vi "modbusTxLoop.vi"(11 "Modbus Port Settings":T1) -> ()   [LabVIEW 2015]
uses:
  DataTypes/ModbusPortSettings.ctl
  DataTypes/TxLoopData.ctl
  DataTypes/TxStates.ctl
  <vilib>/Platform/TimedLoop/XDataNode/timing_clust.ctl
  <vilib>/Platform/TimedLoop/XDataNode/nitl_modes.ctl
  <vilib>/Platform/TimedLoop/XDataNode/wakeup.ctl
  Telemetry/DataTypes/TelemetryUpdateMode.ctl
  <vilib>/rvi/Emulation/niFpgaSctlEmulationGetInTimedLoop.vi
  <vilib>/rvi/Emulation/niFpgaEmulationReportErrorSimple.vi
  <vilib>/rvi/Emulation/niFpgaGetClockAttributes.vi
  <vilib>/rvi/Emulation/niFpgaCriticalErrorInLSC.vi
  <vilib>/rvi/Emulation/niFpgaEmulationIsFPGAContextNoSignature.vi
  <vilib>/rvi/DataTransferAndStorage/Container/Common/niFpgaContainerGetUniqueNameForEmu.vi
  <vilib>/rvi/Memory/Memory_Emulation/niFpgaMemoryEmulationCacheClearOnFirstRun.vi
  <vilib>/rvi/Memory/Memory_Emulation/nirvimemoryEmulationManagerCache_MakeExclusive.vi
  <vilib>/rvi/Memory/Memory_Emulation/niFpgaMemoryEmulationValidateCache.vi
  <vilib>/rvi/Memory/Memory_Emulation/nirvimemoryEmulationManagerCache_InsertValue.vi
  <vilib>/Utility/error.llb/Clear Errors.vi
  <vilib>/rvi/Memory/Memory_Emulation/nirvimemoryEmulationManagerCache_ReleaseExclusive.vi
  <vilib>/rvi/Memory/Memory_Emulation/nirvimemoryEmulationManagerCache_GetValue.vi
  <vilib>/rvi/Memory/Memory_Emulation/nirvimemoryEmulationManagerCache_SetValue.vi
  <vilib>/rvi/Emulation/niFpgaProcessEmulError.vi
  <vilib>/rvi/DataTransferAndStorage/Container/Common/niFpgaContainerExecOnDevCompGetState.vi
  <vilib>/rvi/errors/niFpgaSetErrorForExecOnDevCompSimple.vi
  <vilib>/rvi/eio/common/nirviEmuReportErrorAndStop.vi
  <vilib>/rvi/FIFO/Fifo_Resource/nirvififoEmulationSetSize.vi
  <vilib>/rvi/FIFO/Fifo_Resource/nirviFifoEmulationQueueMgr.vi
  <instcachedir>/0/nirviFifoEmulationQueueMgr_E5CAEC123FF24DC58D834DCA3CDAA9B5.lvgen/nirviFifoEmulationQueueMgr_E5CAEC123FF24DC58D834DCA3CDAA9B5_010.vi
  <vilib>/rvi/FIFO/Fifo_Resource/nirvififoEmulationDetermineInputValidOut.vi
  <vilib>/rvi/FIFO/Fifo_Resource/nirvififoEmulationCreateLock.vi
  <vilib>/rvi/FIFO/Fifo_Resource/nirvififoEmulationObtainLock.vi
  <vilib>/rvi/FIFO/Fifo_Resource/nirvififoEmulationReleaseLock.vi
  <vilib>/rvi/occurrence/nirviWaitOnOccurrenceBase.vi
  <vilib>/rvi/errors/nirviReportUnexpectedCaseInternalError.vi
  <vilib>/rvi/errors/nirviReportUnexpectedCaseInternalError (U32).vi
  <vilib>/rvi/interface/RandomDataEmulation/niFpgaRandomDataHandleErrors.vi
  <vilib>/rvi/eio/common/nirviEmuTemplateMethod_errors.vi
  <vilib>/Platform/TimedLoop/XDataNode/XDataNode.xnode
  <vilib>/rvi/DataTransferAndStorage/Container/XNode/niFpgaContainer.xnode
  <vilib>/rvi/DataTransferAndStorage/Register/Emulation/niFpgaRegisterEmulation.vi
  <vilib>/rvi/FIFO/Fifo_Resource/niFpgaFifoEmulationRefIn.vi
  <vilib>/rvi/DataTransferAndStorage/Register/Emulation/niFpgaRegisterEmulationRefIn.vi
  <vilib>/eio/EIONode/EIONode.xnode
  <vilib>/Platform/TimedLoop/XDataNode/XDNodeRunTimeDep.lvlib
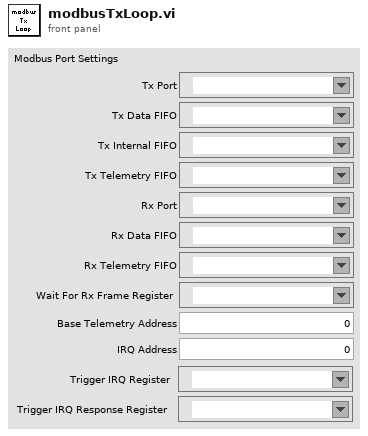
[diagram p1: front panel]
types:
  T1 = typedef "ModbusPortSettings.ctl" = cluster{"Tx Port":refnum<k21>, "Tx Data FIFO":refnum<k21>, "Tx Internal FIFO":refnum<k21>, "Tx Telemetry FIFO":refnum<k21>, "Rx Port":refnum<k21>, "Rx Data FIFO":refnum<k21>, "Rx Telemetry FIFO":refnum<k21>, "Base Telemetry Address":u32, "Wait For Rx Frame Register":refnum<k21>, "IRQ Address":u8, "Trigger IRQ Register":refnum<k21>, "Trigger IRQ Response Register":refnum<k21>}
  T2 = typedef "TxLoopData.ctl" = cluster{"State":T3, "Write Data":u16, "Delay Ticks":u32, "State After Delay":T3, "Bit":u16, "Bytes Sent":u16, "Last IRQ Response":bool}
  T3 = typedef "TxStates.ctl" = enum16{"TryReadInstruction", "Delay", "WriteBits", "WaitForRxFrame", "TriggerIRQ"}
  T4 = typedef "XDNodeRunTimeDep.lvlib/timing_clust.ctl" = cluster{"Expected End [f-1]":u64, "Actual End [f-1]":u64, "Finished Late? [f-1]":bool, "Expected End [i-1]":u64, "Actual End [i-1]":u64, "Finished Late? [i-1]":bool, "Expected Start [i]":u64, "Actual Start [i]":u64, "Expected Start [f]":u64, "Actual Start [f]":u64, "Source Name":string, "Structure Name":string, "Period":i64, "Deadline":i64, "Offset":i64, "Start":i64, "Priority":i32, "Timeout":i32, "Mode":T5, "Wakeup Reason":T6, "Error":errorcluster, "Source Type":string, "Secondary Source Type":string, "Global End Time":u64, "Global Start Time":u64, "Frame Duration":u64, "Iteration Duration":u64, "Assigned CPU":i32, "I/O Scan Engine Mode":u32}
  T5 = typedef "XDNodeRunTimeDep.lvlib/nitl_modes.ctl" = enum32{"No Change", "Process missed periods, maintain original phase", "Discard missed periods, maintain original phase", "Process missed periods, ignore original phase", "Discard missed periods, ignore original phase"}
  T6 = typedef "XDNodeRunTimeDep.lvlib/wakeup.ctl" = enum32{"Normal", "Aborted", "Asynchronous wakeup", "Timing source error", "Timed loop error", "Timeout"}
  T7 = typedef "TelemetryUpdateMode.ctl" = enum8{"NOP", "Set", "Add", "Subtract", "Or"}
  T8 = cluster{"Tx Instruction Type":enum8{"NOP", "WriteByte", "EndOfFrame", "DelayTicks", "DelayMicroseconds", "DelayMilliseconds", "WaitForRxFrame", "TriggerIRQ"}, "Data":u16}
  T9 = enum8{"NOP", "WriteByte", "EndOfFrame", "DelayTicks", "DelayMicroseconds", "DelayMilliseconds", "WaitForRxFrame", "TriggerIRQ"}
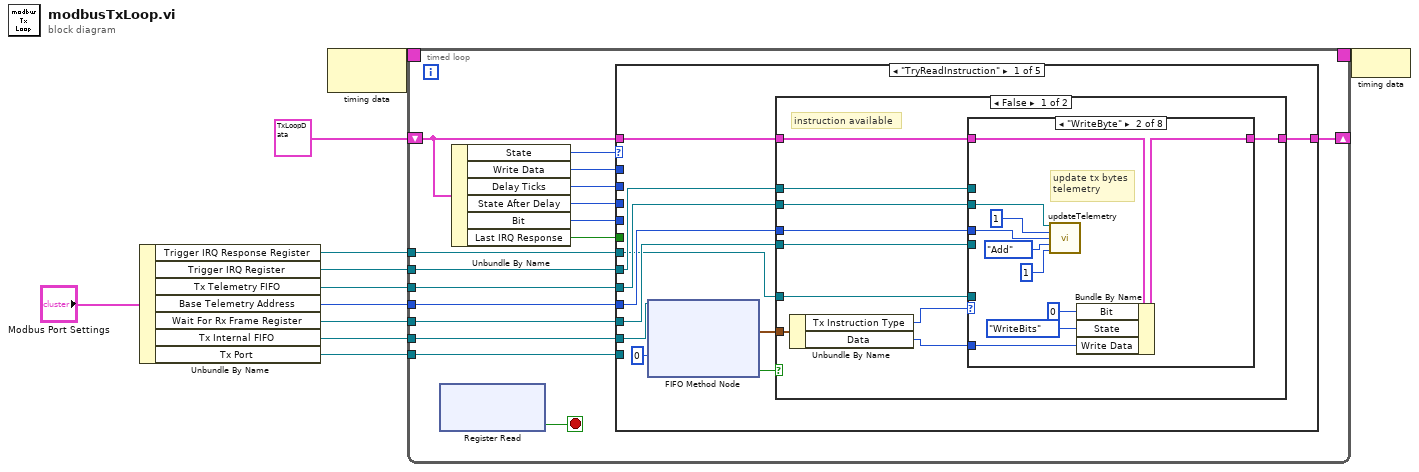
[diagram p0: block diagram]
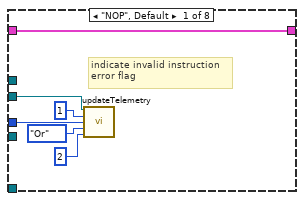
[diagram p2: hidden frame]
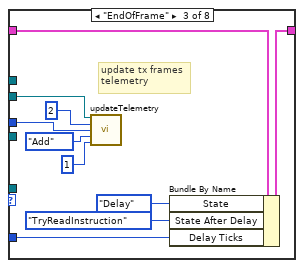
[diagram p3: hidden frame]
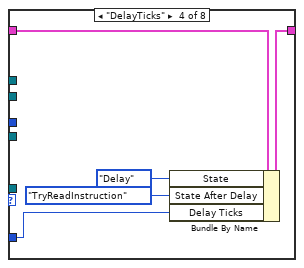
[diagram p4: hidden frame]
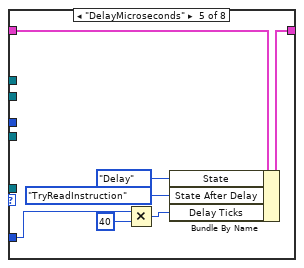
[diagram p5: hidden frame]
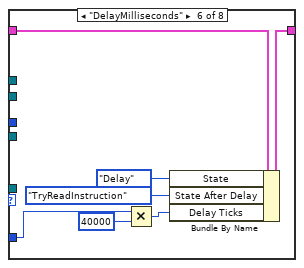
[diagram p6: hidden frame]
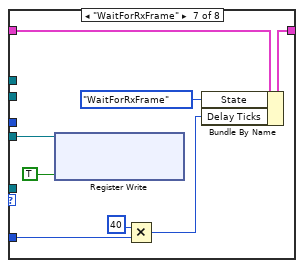
[diagram p7: hidden frame]
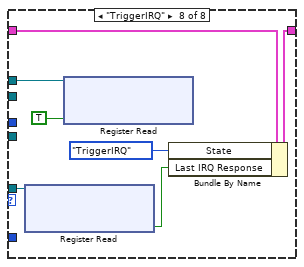
[diagram p8: hidden frame]
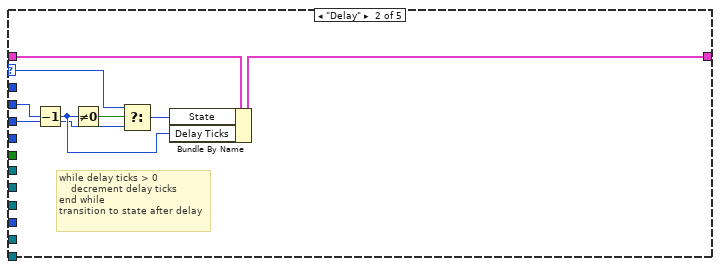
[diagram p10: hidden frame]
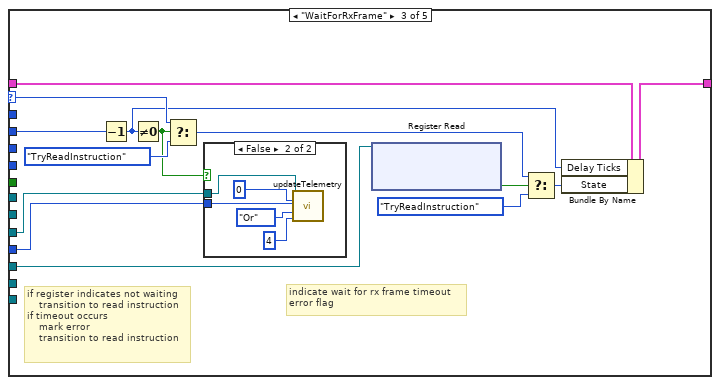
[diagram p11: hidden frame]
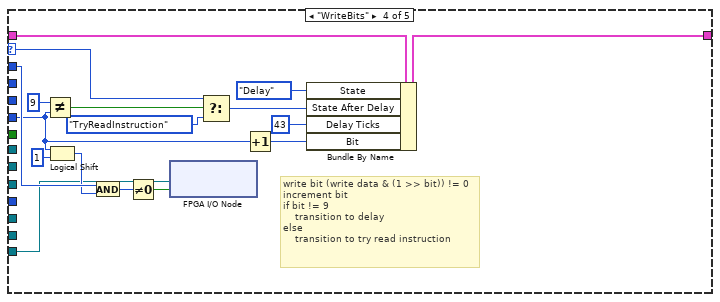
[diagram p13: hidden frame]
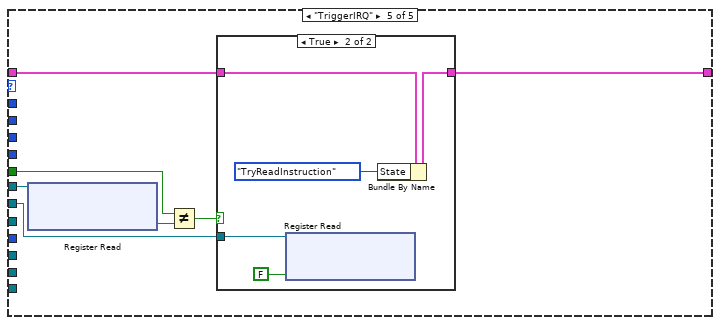
[diagram p14: hidden frame]
diagram:
  n1 = Unbundle By Name("Modbus Port Settings") -> ("Trigger IRQ Response Register"=w9:refnum<k21>, "Trigger IRQ Register"=w8:refnum<k21>, "Tx Telemetry FIFO"=w3:refnum<k21>, "Base Telemetry Address"=w4:u32, "Wait For Rx Frame Register"=w5:refnum<k21>, "Tx Internal FIFO"=w6:refnum<k21>, "Tx Port"=w7:refnum<k21>)
  n2 = node-c288() -> (w11:T4)  [unwired: 1 in]
  n3 = timed-loop {
    shift-right: [w26] -> _
    shift-left: T2 {"State"=enum."TryReadInstruction", "Write Data"=0, "Delay Ticks"=0, "State After Delay"=enum."TryReadInstruction", "Bit"=0, "Bytes Sent"=0, "Last IRQ Response"=FALSE} ("ModbusTxLoop") -> [w25]
    tunnel: w5 -> [w23]
    tunnel: w4 -> [w19]
    tunnel: w3 -> [w17]
    timing: w11 -> [_]
    timing-out: [_] -> w10
    tunnel: w6 -> [w16]
    tunnel: w7 -> [w15]
    tunnel: w8 -> [w14]
    tunnel: w9 -> [w13]
    stop <- w27 stop-if-true
    n4 = xnode ("Register Read")() -> ("Data"=w27:bool)  [unwired: 1 in, 1 out]
    n5 = Unbundle By Name(w25) -> ("State"=w24:T3, "Write Data"=w22:u16, "Delay Ticks"=w21:u32, "State After Delay"=w20:T3, "Bit"=w18:u16, "Last IRQ Response"=w12:bool)
    n6 = case shown="\"TryReadInstruction\"" w24 {
      selector: w24 -> [_ w113 w124 w147 _]
      tunnel: w25 -> [w35 w117 w129 w150 w156]
      tunnel: [w34 w116 w128 w145 w155] -> w26
      tunnel: w23 -> [w32 _ w126 _ _]
      tunnel: w22 -> [_ _ _ w152 _]
      tunnel: w21 -> [_ w115 w125 _ _]
      tunnel: w20 -> [_ w110 _ _ _]
      tunnel: w19 -> [w31 _ w118 _ _]
      tunnel: w18 -> [_ _ _ w140 _]
      tunnel: w17 -> [w30 _ w119 _ _]
      tunnel: w16 -> [w33 _ _ _ _]
      tunnel: w15 -> [_ _ _ w137 _]
      tunnel: w14 -> [w29 _ _ _ w154]
      tunnel: w13 -> [w28 _ _ _ w160]
      tunnel: w12 -> [_ _ _ _ w158]
      frame "TryReadInstruction" {
        n7 = xnode ("FIFO Method Node")("Timeout"=0, "FIFO In"=w33) -> ("Element"=w36:T8, "Timed Out?"=w37:bool)  [unwired: 1 out]
        n8 = case shown="False" w37 {
          tunnel: w36 -> [w44 _]
          tunnel: w35 -> [w48 w109]
          tunnel: [w47 w109] -> w34
          tunnel: w31 -> [w46 _]
          tunnel: w30 -> [w45 _]
          tunnel: w32 -> [w41 _]
          tunnel: w29 -> [w40 _]
          tunnel: w28 -> [w39 _]
          frame False {
            # "instruction available"
            # "instruction available"
            n9 = Unbundle By Name(w44) -> ("Tx Instruction Type"=w42:T9, "Data"=w43:u16)
            n10 = case shown="\"WriteByte\"" w42 {
              tunnel: w43 -> [_ w63 w73 w75 w82 w89 w96 _]
              tunnel: w48 -> [w54 w64 w74 w79 w86 w93 w101 w108]
              tunnel: [w54 w62 w71 w77 w84 w91 w100 w107] -> w47
              tunnel: w46 -> [w50 w56 w66 _ _ _ _ _]
              tunnel: w45 -> [w49 w55 w65 _ _ _ _ _]
              tunnel: w41 -> [_ _ _ _ _ _ w97 _]
              tunnel: w40 -> [_ _ _ _ _ _ _ w105]
              tunnel: w39 -> [_ _ _ _ _ _ _ w103]
              frame "NOP", Default {
                # "indicate invalid instruction\nerror flag"
                # "nop"
                n11 = call "updateTelemetry.vi"("Telemetry FIFO"=w49, "Address Offset"=u32 1 ("x"), "Base Address"=w50, "Telemetry Update Mode"=TelemetryUpdateMode."Or", "Data"=u32 2) -> ()  [unwired: 11 in]
              }
              frame "WriteByte" {
                # "update tx bytes\ntelemetry"
                # "transition to write bits"
                n12 = call "updateTelemetry.vi"("Telemetry FIFO"=w55, "Address Offset"=u32 1 ("x"), "Base Address"=w56, "Telemetry Update Mode"=TelemetryUpdateMode."Add", "Data"=u32 1) -> ()  [unwired: 11 in]
                n13 = Bundle By Name(cluster=w64, "Bit"=u16 0, "State"=TxStates."WriteBits", "Write Data"=w63) -> (w62:T2)
              }
              frame "EndOfFrame" {
                # "update tx frames\ntelemetry"
                # "transition to delay"
                n14 = call "updateTelemetry.vi"("Telemetry FIFO"=w65, "Address Offset"=u32 2 ("x"), "Base Address"=w66, "Telemetry Update Mode"=TelemetryUpdateMode."Add", "Data"=u32 1) -> ()  [unwired: 11 in]
                n15 = Bundle By Name(cluster=w74, "State"=TxStates."Delay" ("TransmitStates"), "State After Delay"=TxStates."TryReadInstruction" ("TransmitStates"), "Delay Ticks"=w73) -> (w71:T2)
              }
              frame "DelayTicks" {
                # "transition to delay"
                n16 = Bundle By Name(cluster=w79, "State"=TxStates."Delay" ("TransmitStates"), "State After Delay"=TxStates."TryReadInstruction" ("TransmitStates"), "Delay Ticks"=w75) -> (w77:T2)
              }
              frame "DelayMicroseconds" {
                # "transition to delay"
                n17 = Multiply(x=w82, y=u16 40) -> (x*y=w80:u16)
                n18 = Bundle By Name(cluster=w86, "State"=TxStates."Delay" ("TransmitStates"), "State After Delay"=TxStates."TryReadInstruction" ("TransmitStates"), "Delay Ticks"=w80) -> (w84:T2)
              }
              frame "DelayMilliseconds" {
                # "transition to delay"
                n19 = Multiply(x=w89, y=u16 40000) -> (x*y=w87:u16)
                n20 = Bundle By Name(cluster=w93, "State"=TxStates."Delay" ("TransmitStates"), "State After Delay"=TxStates."TryReadInstruction" ("TransmitStates"), "Delay Ticks"=w87) -> (w91:T2)
              }
              frame "WaitForRxFrame" {
                # "transition to delay"
                n21 = xnode ("Register Write")("Data"=TRUE, "Register In"=w97) -> ()  [unwired: 1 out]
                n22 = Multiply(x=u16 40, y=w96) -> (x*y=w95:u16)
                n23 = Bundle By Name(cluster=w101, "State"=TxStates."WaitForRxFrame" ("TransmitStates"), "Delay Ticks"=w95) -> (w100:T2)
              }
              frame "TriggerIRQ" {
                # "transition to delay"
                n24 = xnode ("Register Read")("Register In"=w103) -> ("Data"=w102:bool)  [unwired: 1 out]
                n25 = xnode ("Register Read")("Data"=TRUE, "Register In"=w105) -> ()  [unwired: 1 out]
                n26 = Bundle By Name(cluster=w108, "State"=TxStates."TriggerIRQ", "Last IRQ Response"=w102) -> (w107:T2)
              }
            }
          }
          frame True {
            # "no instruction available"
            # "no instruction available"
          }
        }
      }
      frame "Delay" {
        # "while delay ticks > 0\n    decrement delay ticks\nend while\ntransition to state after delay"
        n27 = Decrement(x=w115) -> (x-1=w111:u32)
        n28 = Not Equal To 0?(x=w111) -> (x != 0?=w114:bool)
        n29 = Select(t=w113, s=w114, f=w110) -> (s? t:f=w112:T3)
        n30 = Bundle By Name(cluster=w117, "State"=w112, "Delay Ticks"=w111) -> (w116:T2)
      }
      frame "WaitForRxFrame" {
        # "indicate wait for rx frame timeout\nerror flag"
        # "if register indicates not waiting\n    transition to read instruction\nif timeout occurs\n    mark error\n    transition to read instruction"
        n31 = Decrement(x=w125) -> (x-1=w121:u32)
        n32 = Not Equal To 0?(x=w121) -> (x != 0?=w120:bool)
        n33 = Select(t=w124, s=w120, f=TxStates."TryReadInstruction") -> (s? t:f=w123:T3)
        n34 = case shown="False" w120 {
          tunnel: w119 -> [_ w135]
          tunnel: w118 -> [_ w134]
          frame True {
          }
          frame False {
            n35 = call "updateTelemetry.vi"("Telemetry FIFO"=w135, "Address Offset"=u32 0 ("x"), "Base Address"=w134, "Telemetry Update Mode"=TelemetryUpdateMode."Or", "Data"=u32 4) -> ()  [unwired: 11 in]
          }
        }
        n36 = xnode ("Register Read")("Register In"=w126) -> ("Data"=w131:bool)  [unwired: 1 out]
        n37 = Select(t=w123, s=w131, f=TxStates."TryReadInstruction") -> (s? t:f=w127:T3)
        n38 = Bundle By Name(cluster=w129, "Delay Ticks"=w121, "State"=w127) -> (w128:T2)
      }
      frame "WriteBits" {
        # "write bit (write data & (1 >> bit)) != 0\nincrement bit\nif bit != 9\n    transition to delay\nelse\n    transition to try read instruction"
        n39 = Not Equal?(x=u16 9, y=w140) -> (x != y?=w139:bool)
        n40 = Logical Shift(y=w140, x=u16 1) -> (x << y=w142:u16)
        n41 = And(x=w152, y=w142) -> (x .and. y?=w153:u16)
        n42 = Not Equal To 0?(x=w153) -> (x != 0?=w151:bool)
        n43 = xnode "FPGA I/O Node"("I/O Item"=w151, "FPGA I/O In"=w137) -> ()  [unwired: 1 out]
        n44 = Select(t=w147, s=w139, f=TxStates."TryReadInstruction" ("TransmitStates")) -> (s? t:f=w149:T3)
        n45 = Increment(x=w140) -> (x+1=w144:u16)
        n46 = Bundle By Name(cluster=w150, "State"=TxStates."Delay" ("TransmitStates"), "State After Delay"=w149, "Delay Ticks"=u16 43, "Bit"=w144) -> (w145:T2)
      }
      frame "TriggerIRQ" {
        n47 = xnode ("Register Read")("Register In"=w160) -> ("Data"=w159:bool)  [unwired: 1 out]
        n48 = Not Equal?(x=w158, y=w159) -> (x != y?=w157:bool)
        n49 = case shown="True" w157 {
          tunnel: w156 -> [w161 w166]
          tunnel: [w161 w165] -> w155
          tunnel: w154 -> [_ w164]
          frame False {
          }
          frame True {
            n50 = xnode ("Register Read")("Data"=FALSE, "Register In"=w164) -> ()  [unwired: 1 out]
            n51 = Bundle By Name(cluster=w166, "State"=TxStates."TryReadInstruction") -> (w165:T2)
          }
        }
      }
    }
  }
  n52 = node-c288(w10) -> ()
